vi "ConvertByteArrToStr.vi"(11 "Data":u8[](array[numeric])) -> (2 "Hex Data":string, 3 "Hex String":string)   [LabVIEW 2018, in "Library-DataConvert.lvlib"]
uses:
  Library-DataConvert.lvlib
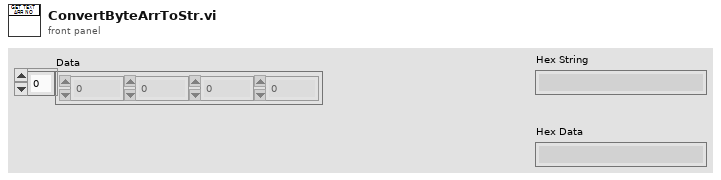
[diagram p1: front panel]
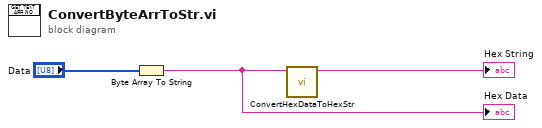
[diagram p0: block diagram]
diagram:
  n1 = Byte Array To String(unsigned byte array="Data") -> (string=w1:string)
  "Hex Data" <- w1
  n2 = call "ConvertHexDataToHexStr.vi"("hex data(not string)"=w1) -> ("string-hex"=→"Hex String":string)  [unwired: 10 in]
